vi "Get move string.vi"(7 "Position":refnum<class "Position.lvclass">, 8 "error in (no error)":errorcluster, 11 "Move in":refnum<class "Move.lvclass">) -> (0 "error out":errorcluster, 2 "Move string":string, 3 "Move out":refnum<class "Move.lvclass">)   [LabVIEW 2016, in "Chesslib.lvlib" / "Move.lvclass"]
uses:
  Move.lvclass
  Position/Position.lvclass
  Move.lvclass/Move.ctl
  Pieces/Piece/Piece.lvclass
  Chesslib.lvlib
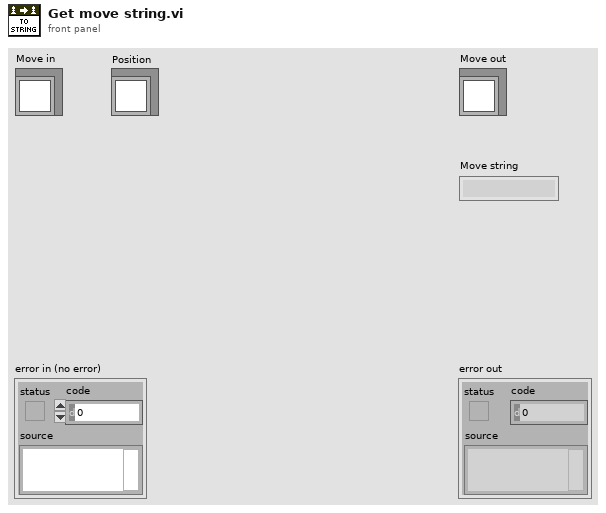
[diagram p1: front panel]
types:
  T1 = typedef "Chesslib.lvlib/Square.ctl" = cluster{"File":T2, "Rank":T3}
  T2 = typedef "Chesslib.lvlib/File.ctl" = enum8{"a", "b", "c", "d", "e", "f", "g", "h"}
  T3 = typedef "Chesslib.lvlib/Rank.ctl" = enum8{"1", "2", "3", "4", "5", "6", "7", "8"}
  T4 = typedef "Chesslib.lvlib/Piece type.ctl" = enum16{"Pawn", "Bishop", "Knight", "Rook", "Queen", "King"}
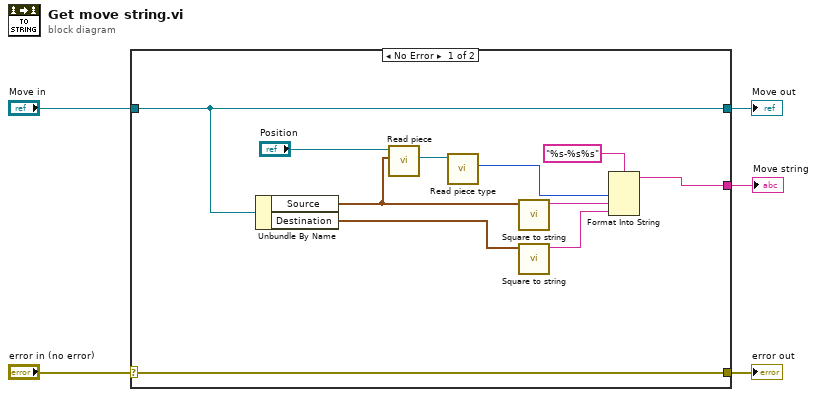
[diagram p0: block diagram]
diagram:
  n1 = case shown="No Error" "error in (no error)" {
    selector: "error in (no error)" -> [w16 w18]
    tunnel: [w16 w18] -> w4
    tunnel: [w15 w17] -> w2
    tunnel: "Move in" -> [w15 w17]
    tunnel: [w10 _] -> w1
    frame No Error {
      n2 = Unbundle By Name(w15) -> ("Source"=w8:T1, "Destination"=w14:T1)
      n3 = call "Read piece.vi"("Square"=w8, "Position in"="Position") -> ("Piece"=w7:refnum<class "Piece.lvclass">)  [unwired: 7 in, 2 out]
      n4 = call-dynamic "Read piece type.vi"("Piece in"=w7) -> ("Piece type"=w6:T4)  [unwired: 10 in]
      n5 = call "Square to string.vi"("Square"=w8) -> ("Square string"=w13:string)  [unwired: 10 in]
      n6 = call "Square to string.vi"("Square"=w14) -> ("Square string"=w12:string)  [unwired: 10 in]
      n7 = Format Into String(format string="%s-%s%s", w6, w13, w12) -> (resulting string=w10:string)  [unwired: 2 in, 1 out]
    }
    frame Error {
    }
  }
  "error out" <- w4
  "Move out" <- w2
  "Move string" <- w1
